vi "Int64Array Create (Dimensions).vi"(8 "error in (no error)":errorcluster, 10 "Array dimensions":i32[](array[numeric]), 11 "I64 array in":i64[](array[numeric])) -> (0 "error out":errorcluster, 3 "Int64Array DVR out":refnum<data-value>)   [LabVIEW 2010, in "MDSplus.lvlib"]
uses:
  <vilib>/MDSplus/Library/MDSplus.lvlib
  <vilib>/MDSplus/Classes/Data_Class/Array_Class/Int64Array_Class/Int64Array.lvclass
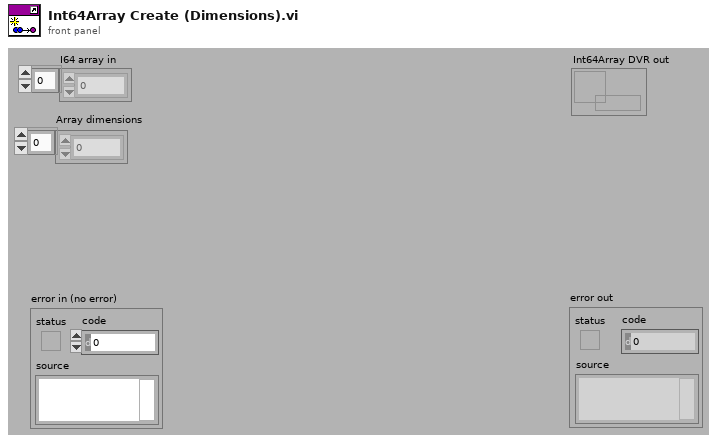
[diagram p1: front panel]
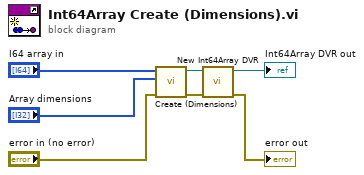
[diagram p0: block diagram]
diagram:
  n1 = call <vilib>:"Create (Dimensions).vi"("error in (no error)"="error in (no error)", "Dimensions"="Array dimensions", "I64 array in"="I64 array in") -> ("error out"=w4:errorcluster, "Int64Array out"=w5:refnum<class "Int64Array.lvclass">)  [unwired: 7 in]
  n2 = call <vilib>:"New Int64Array DVR.vi"("error in (no error)"=w4, "Int64Array in"=w5) -> ("error out"=→"error out":errorcluster, "Int64Array DVR out"=→"Int64Array DVR out":refnum<data-value>)  [unwired: 8 in]
